vi "select_change.vi"(10 "Value in":u16, 11 "Ring in":refnum<vi>) -> (0 "Ring out":refnum<vi>, 3 "selected":bool)   [LabVIEW 2015]
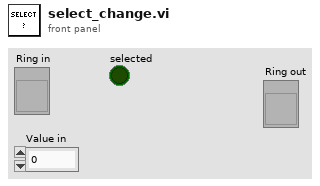
[diagram p1: front panel]
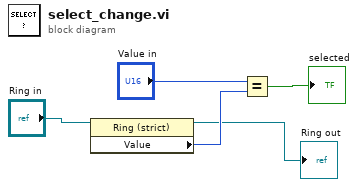
[diagram p0: block diagram]
diagram:
  n1 = property on="Property Node" class="Ring (strict)"(reference="Ring in") -> (reference out=→"Ring out":refnum<vi>, "Value"=w2:u16)  [unwired: 1 in, 1 out]
  n2 = Equal?(x="Value in", y=w2) -> (x = y?=→"selected":bool)
